vi "Add Control Caption.vi"(8 "error in (no error)":errorcluster, 11 "Control Info in":refnum<class "Control Info.lvclass">) -> (0 "error out":errorcluster, 3 "Control Info out":refnum<class "Control Info.lvclass">)   [LabVIEW 2017, in "Localization.lvlib" / "Control Info.lvclass"]
doc: "VI for override that is supposed to do go throgh and create the Caption for the specific VI. Then the caption is set as visible and the label is hidden.\n\nChoose Movement Consulting, LLC"
uses:
  Control Info.lvclass
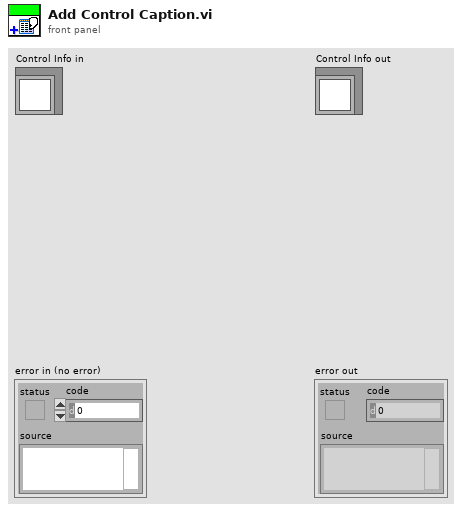
[diagram p1: front panel]
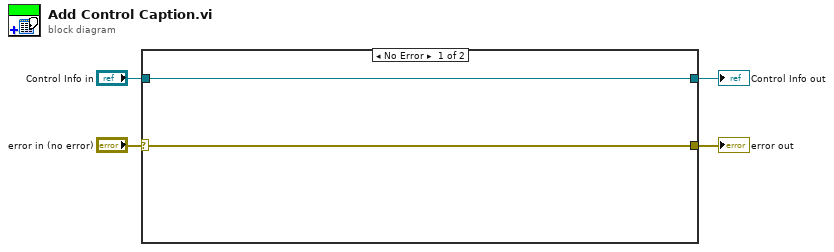
[diagram p0: block diagram]
diagram:
  n1 = case shown="No Error" "error in (no error)" {
    selector: "error in (no error)" -> [w5 w8]
    tunnel: [w5 w8] -> w3
    tunnel: [w6 w7] -> w1
    tunnel: "Control Info in" -> [w6 w7]
    frame No Error {
    }
    frame Error {
    }
  }
  "error out" <- w3
  "Control Info out" <- w1
